vi "Create User Event - Stop.vi"(8 "error in (no error)":errorcluster) -> (0 "error out":errorcluster, 3 "User Events":T1)   [LabVIEW 2020, in "User Event - Stop.lvlib"]
doc: "Create a boolean user events that will be used to stop the event loop from the message handling loop and to manage error events."
uses:
  User Event - Stop.lvlib
  Controls/Events_User.ctl
  Controls/Events_Boolean.ctl
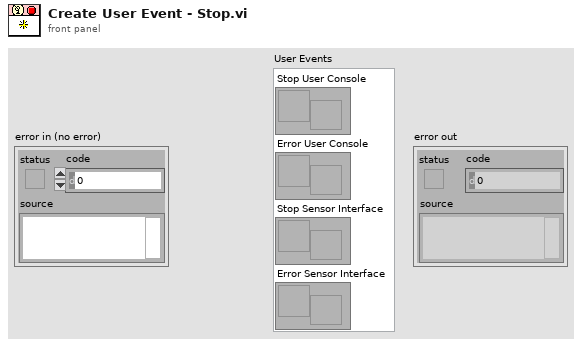
[diagram p1: front panel]
types:
  T1 = typedef "Events_User.ctl" = cluster{"Stop User Console":refnum<user-event>, "Error User Console":refnum<user-event>, "Stop Sensor Interface ":refnum<user-event>, "Error Sensor Interface":refnum<user-event>}
  T2 = typedef "Events_Boolean.ctl" = cluster{"Stop User Console":bool, "Error User Console":bool, "Stop Sensor Interface":bool, "Error Sensor Interface":bool}
  T3 = cluster{"[0]":refnum<user-event>, "[1]":refnum<user-event>, "[2]":refnum<user-event>, "[3]":refnum<user-event>}
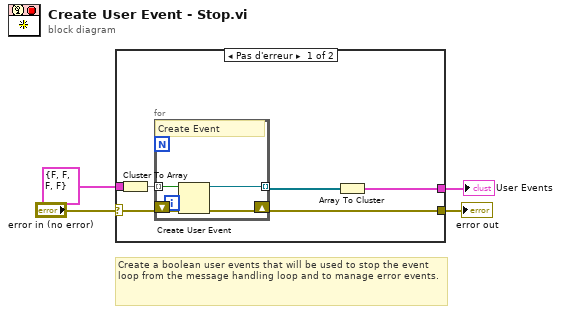
[diagram p0: block diagram]
diagram:
  # "Create a boolean user events that will be used to stop the event loop from the message handling loop and to manage error events."
  n1 = case shown="Pas d'erreur" "error in (no error)" {
    selector: "error in (no error)" -> [w9 w15]
    tunnel: [w5 _] -> w2
    tunnel: [w10 w15] -> w4
    tunnel: T2 {"Stop User Console"=FALSE, "Error User Console"=FALSE, "Stop Sensor Interface"=FALSE, "Error Sensor Interface"=FALSE} ("Events_Bool") -> [w8 _]
    frame No Error {
      n2 = Cluster To Array(cluster=w8) -> (array=w7:bool[])
      n3 = for {
        shift-right: [w14] -> w10
        shift-left: w9 -> [w13]
        tunnel: w7 -> [w12] mode=indexing
        tunnel: [w11] -> w6 mode=indexing
        # "Create Event"
        n4 = Create User Event(user event datatype=w12, error in=w13) -> (user event=w11:refnum<user-event>, error out=w14:errorcluster)
      }
      n5 = Array To Cluster(array=w6) -> (cluster=w5:T3)
    }
    frame Error {
    }
  }
  "error out" <- w4
  "User Events" <- w2
